vi "Sampling Rate.vi"(4 "input a1":dbl, 6 "input y1":dbl, 7 "T(0-1)":dbl(slide) scale=0.0..1.0, 8 "input x1":dbl, 9 "input a0":dbl, 10 "input y0":dbl, 11 "input x0":dbl) -> (0 "GoalT/F":bool, 1 "a_output":dbl, 2 "y_output":dbl, 3 "x_output":dbl)   [LabVIEW 2019]
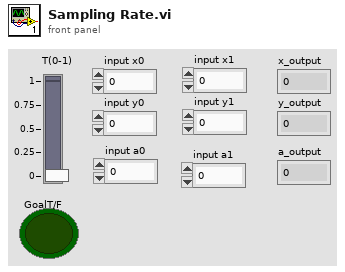
[diagram p1: front panel]
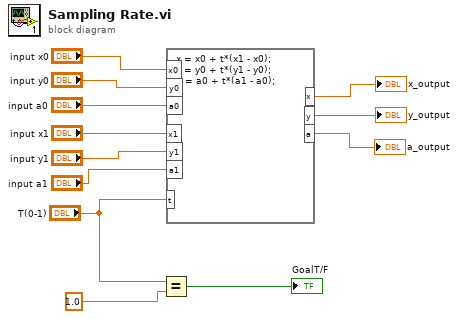
[diagram p0: block diagram]
diagram:
  n1 = Equal?(x="T(0-1)", y=1.0) -> (x = y?=→"GoalT/F":bool)
  n2 = formula code="x = x0 + t*(x1 - x0);\ny = y0 + t*(y1 - y0);\na = a0 + t*(a1 - a0);"("x0"="input x0", "y0"="input y0", "a0"="input a0", "x1"="input x1", "y1"="input y1", "a1"="input a1", "t"="T(0-1)") -> ("x"=→"x_output":dbl, "y"=→"y_output":dbl, "a"=→"a_output":dbl)
